vi "Talker.vi"(0 "Subtract in":refnum<class "Subtract.lvclass">, 5 "Subpanel Ref":refnum<vi>, 11 "Error In":errorcluster) -> (4 "Subtract out":refnum<class "Subtract.lvclass">, 15 "Error Out":errorcluster)   [LabVIEW 2020, in "Subtract.lvclass"]
doc: "Method to call the UI Method. This will pass the object to the UI Method which will do the operation and return the object to the main vi."
uses:
  Subtract.lvclass
  UI.vi
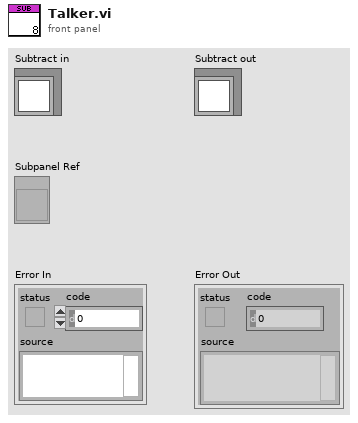
[diagram p1: front panel]
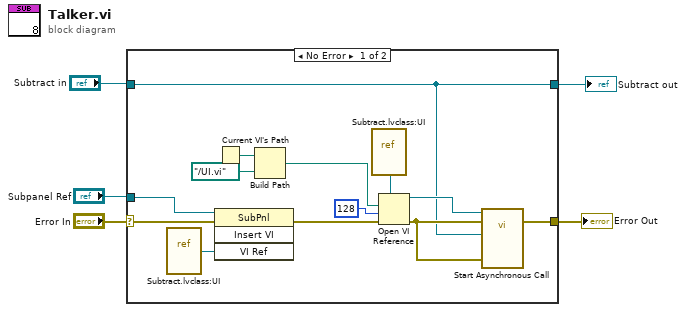
[diagram p0: block diagram]
diagram:
  n1 = case shown="No Error" "Error In" {
    selector: "Error In" -> [w16 w20]
    tunnel: [w12 w20] -> w4
    tunnel: [w11 w19] -> w2
    tunnel: "Subtract in" -> [w11 w19]
    tunnel: "Subpanel Ref" -> [w14 _]
    frame No Error {
      n2 = vi-ref "Subtract.lvclass:UI.vi"() -> (w10:refnum<vi>)
      n3 = invoke on="Invoke Node" class="SubPnl" method="Insert VI"(reference=w14, error in=w16, "VI Ref"=w10) -> (error out=w15:errorcluster)  [unwired: 1 in, 3 out]
      n4 = Current VI's Path() -> (path=w7:path)
      n5 = Build Path(base path=w7, name or relative path=path "../UI.vi") -> (appended path=w6:path)
      n6 = vi-ref "Subtract.lvclass:UI.vi"() -> (w9:refnum<vi>)
      n7 = Open VI Reference(type specifier VI Refnum (for type only)=w9, vi path=w6, options=128, error in (no error)=w15) -> (vi reference=w13:refnum<vi>, error out=w18:errorcluster)  [unwired: 2 in]
      n8 = call-by-ref "Start Asynchronous Call"(reference=w13, error in=w18, "Subtract in"=w11, "Error In"=w18) -> (error out=w12:errorcluster)  [unwired: 11 in, 4 out]
    }
    frame Error {
    }
  }
  "Subtract out" <- w2
  "Error Out" <- w4
